vi "Class to Variant.vi"(8 "error in (no error)":errorcluster, 10 "Data in":variant, 11 "VIPB Build Node in":refnum<class "VIPB Build Node.lvclass">) -> (0 "error out":errorcluster, 1 "Serialized Object Name":string, 2 "Data Out":variant, 3 "VIPB Build Node out":refnum<class "VIPB Build Node.lvclass">)   [LabVIEW 2014, in "VIPB Build Node.lvclass"]
uses:
  VIPB Build Node.lvclass
  Shared/Controls/VIPB Build - STYP.ctl
  VIPB Build Node.lvclass/VIPB Build Node.ctl
  Classes/Build Job/Build Job.lvclass
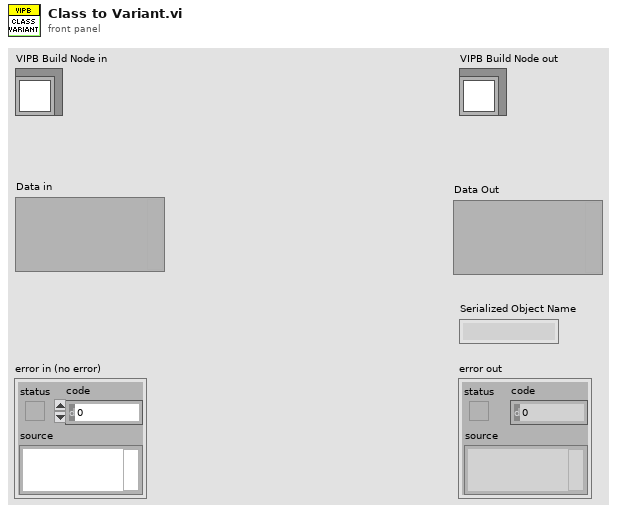
[diagram p1: front panel]
types:
  T1 = typedef "VIPB Build - STYP.ctl" = cluster{"VIPB Path":string, "Install after build":bool, "LabVIEW Version":string}
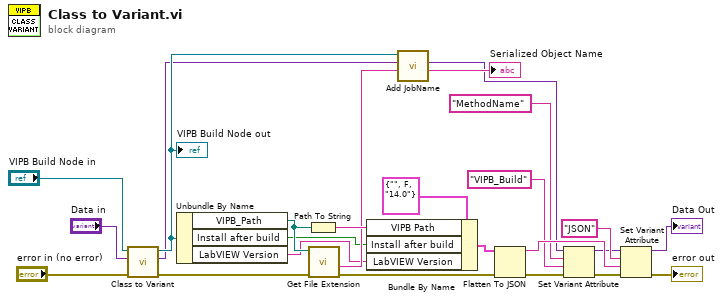
[diagram p0: block diagram]
diagram:
  n1 = call-parent "Class to Variant.vi"("error in (no error)"="error in (no error)", "Data in"="Data in", "Build Job in"="VIPB Build Node in") -> ("error out"=w7:errorcluster, "Data Out"=w4:variant, "Build Job out"=w9:refnum<class "VIPB Build Node.lvclass">)  [unwired: 5 in, 1 out]
  "VIPB Build Node out" <- w9
  n2 = Unbundle By Name(w9) -> ("VIPB_Path"=w8:path, "Install after build"=w2:bool, "LabVIEW Version"=w1:string)
  n3 = Path To String(path=w8) -> (string=w14:string)
  n4 = call <vilib>:"Get File Extension.vi"("error in (no error)"=w7, "file"=w8) -> ("error out"=w6:errorcluster, "filename without extension"=w10:string)  [unwired: 6 in, 2 out]
  n5 = Bundle By Name(cluster=T1 {"VIPB Path"="", "Install after build"=FALSE, "LabVIEW Version"="14.0"} ("VIPB Build"), "VIPB Path"=w14, "Install after build"=w2, "LabVIEW Version"=w1) -> (w16:T1)
  n6 = call "Add JobName.vi"("Job Target"=w10, "Data in"=w4, "Build Job in"=w9) -> ("Job Name"=→"Serialized Object Name":string, "Data Out"=w3:variant)  [unwired: 7 in]
  n7 = Flatten To JSON(anything=w16, error in (no error)=w6) -> (JSON string=w21:string, 11:w22:errorcluster)  [unwired: 1 in]
  n8 = Set Variant Attribute(Variant=w3, name="MethodName", value="VIPB_Build", error in=w22) -> (Variant out=w11:variant, error out=w17:errorcluster)  [unwired: 1 out]
  n9 = Set Variant Attribute(Variant=w11, name="JSON" ("Name"), value=w21, error in=w17) -> (Variant out=→"Data Out":variant, error out=→"error out":errorcluster)  [unwired: 1 out]
